vi "Error.GetError.vi"(11 "Msg":u8[](array[numeric])) -> (3 "error out":errorcluster)   [LabVIEW 2027, in "VS Inline Async API.lvlib"]
uses:
  VS Inline Async API.lvlib
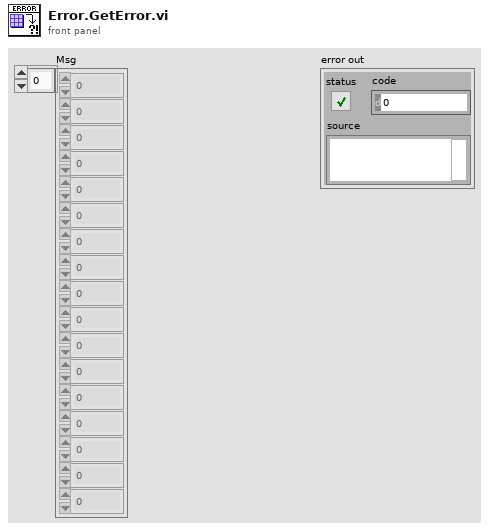
[diagram p1: front panel]
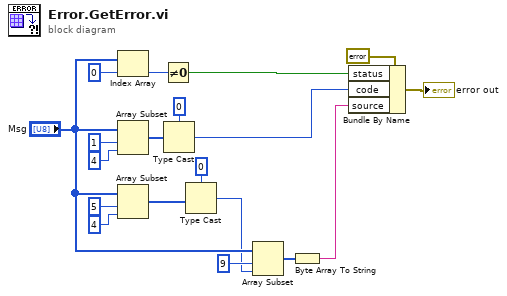
[diagram p0: block diagram]
diagram:
  n1 = Index Array(array="Msg", index=0) -> (element=w6:u8)
  n2 = Array Subset(array="Msg", index=1, length=4) -> (w11:u8[])
  n3 = Array Subset(array="Msg", index=5, length=4) -> (w12:u8[])
  n4 = Not Equal To 0?(x=w6) -> (x != 0?=w4:bool)
  n5 = Type Cast(type=0 ("code"), x=w11) -> (*(type *) &x=w3:i32)
  n6 = Type Cast(type=0 ("length"), x=w12) -> (*(type *) &x=w8:i32)
  n7 = Array Subset(array="Msg", index=9, length=w8) -> (w7:u8[])
  n8 = Byte Array To String(unsigned byte array=w7) -> (string=w2:string)
  n9 = Bundle By Name(cluster=errorcluster {"status"=FALSE, "code"=0, "source"=""} ("error in"), "status"=w4, "code"=w3, "source"=w2) -> (→"error out":errorcluster)
